vi "testUtilitieswithSeparatedSource.vi"(8 "error in (no error)":errorcluster, 11 "testStateMachineUtilities in":refnum<class "testStateMachineUtilities.lvclass">) -> (0 "error out":errorcluster, 3 "testStateMachineUtilities out":refnum<class "testStateMachineUtilities.lvclass">)   [LabVIEW 2020, in "testStateMachineUtilities.lvclass"]
uses:
  testStateMachineUtilities.lvclass
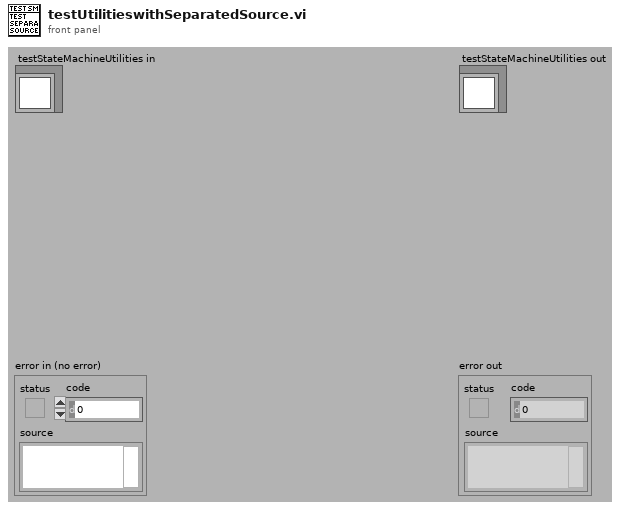
[diagram p1: front panel]
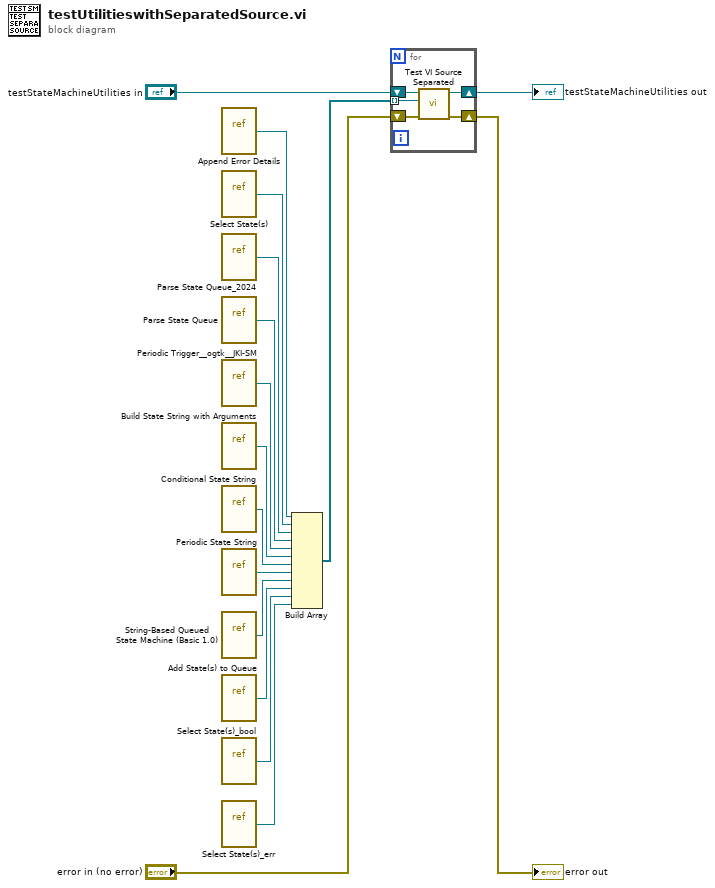
[diagram p0: block diagram]
diagram:
  n1 = vi-ref "Append Error Details.vi"() -> (w13:refnum<vi>)
  n2 = vi-ref "Select State(s).vi"() -> (w12:refnum<vi>)
  n3 = vi-ref "Parse State Queue_2024.vi"() -> (w11:refnum<vi>)
  n4 = vi-ref "Parse State Queue.vi"() -> (w10:refnum<vi>)
  n5 = vi-ref "Periodic Trigger__ogtk__JKI-SM.vi"() -> (w9:refnum<vi>)
  n6 = vi-ref "Build State String with Arguments.vi"() -> (w8:refnum<vi>)
  n7 = vi-ref "Conditional State String.vi"() -> (w7:refnum<vi>)
  n8 = vi-ref "Periodic State String.vi"() -> (w6:refnum<vi>)
  n9 = vi-ref "String-Based Queued State Machine (Basic 1.0).vi"() -> (w5:refnum<vi>)
  n10 = vi-ref "Add State(s) to Queue.vi"() -> (w4:refnum<vi>)
  n11 = vi-ref "Select State(s)_bool.vi"() -> (w3:refnum<vi>)
  n12 = vi-ref "Select State(s)_err.vi"() -> (w2:refnum<vi>)
  n13 = Build Array(w13, w12, w11, w10, w9, w8, w7, w6, w5, w4, w3, w2) -> (w1:refnum<vi>[])
  n14 = for {
    shift-right: [w21] -> w16
    shift-left: "testStateMachineUtilities in" -> [w22]
    shift-right: [w20] -> w15
    shift-left: "error in (no error)" -> [w19]
    tunnel: w1 -> [w18] mode=indexing
    n15 = call "Test VI Source Separated.vi"("error in (no error)"=w19, "VI Refnum"=w18, "testStateMachineUtilities in"=w22) -> ("error out"=w20:errorcluster, "testStateMachineUtilities out"=w21:refnum<class "testStateMachineUtilities.lvclass">)  [unwired: 7 in]
  }
  "error out" <- w15
  "testStateMachineUtilities out" <- w16
